vi "DeQ Valve Transfer State.vi"(8 "error in (no error)":errorcluster, 11 "Syringe Line in":refnum<class "Syringe Line.lvclass">) -> (0 "error out":errorcluster, 1 "timed out?":bool, 2 "State":u16, 3 "Syringe Line out":refnum<class "Syringe Line.lvclass">)   [LabVIEW 2015, in "cRIO-Carbondioxide.lvlib" / "CO2-Actor.lvlib" / "Syringe Line.lvclass"]
uses:
  Syringe Line.lvclass
  Syringe Line.lvclass/Syringe Line.ctl
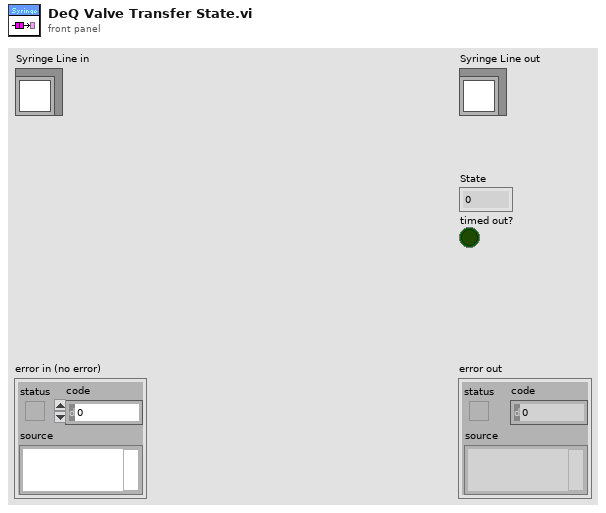
[diagram p1: front panel]
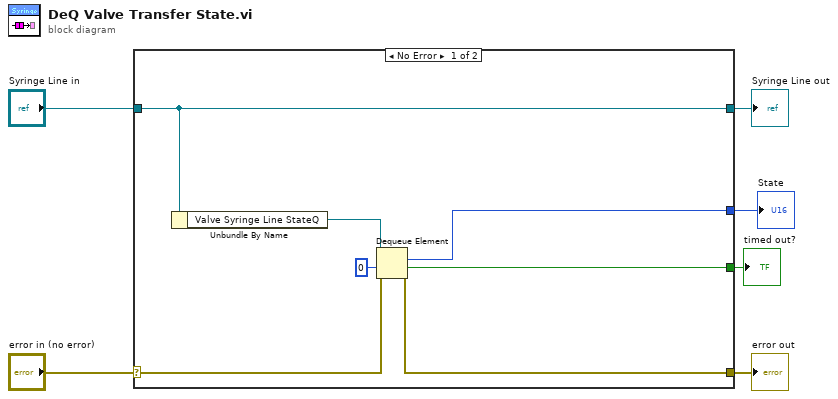
[diagram p0: block diagram]
diagram:
  n1 = case shown="No Error" "error in (no error)" {
    selector: "error in (no error)" -> [w10 w15]
    tunnel: [w9 w15] -> w5
    tunnel: [w13 w14] -> w3
    tunnel: "Syringe Line in" -> [w13 w14]
    tunnel: [w8 _] -> w2
    tunnel: [w7 _] -> w1
    frame No Error {
      n2 = Unbundle By Name(w13) -> ("Valve Syringe Line StateQ"=w12:refnum<queue>)
      n3 = Dequeue Element(queue=w12, timeout in ms (-1)=0, error in (no error)=w10) -> (element=w8:u16, timed out?=w7:bool, error out=w9:errorcluster)  [unwired: 1 out]
    }
    frame Error {
    }
  }
  "error out" <- w5
  "Syringe Line out" <- w3
  "State" <- w2
  "timed out?" <- w1
